vi "4p1_HW_Task2_gamagetd.vi"() -> ()   [LabVIEW 2016]
panel:
  out "Temperature T in C":dbl
  in  "Rois the resistance associated with the reference temperature in Ohm":dbl
  in  "Resistance r in Ohm":dbl
  in  "T-0 a reference temperature (in C)":dbl
  in  "ßis a thermal property of the materials (in K)":dbl
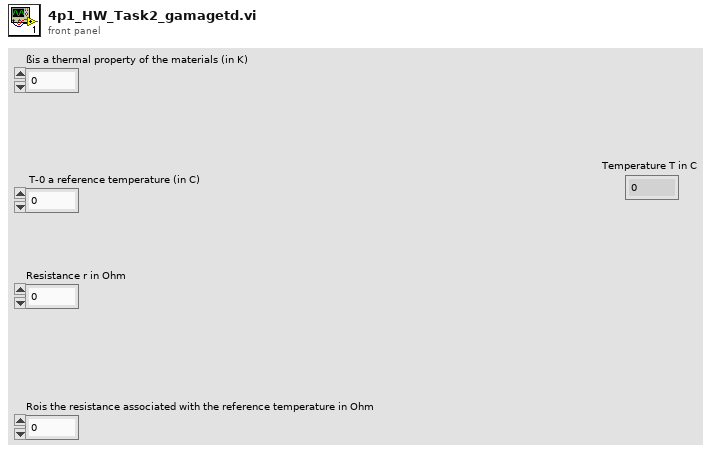
[diagram p1: front panel]
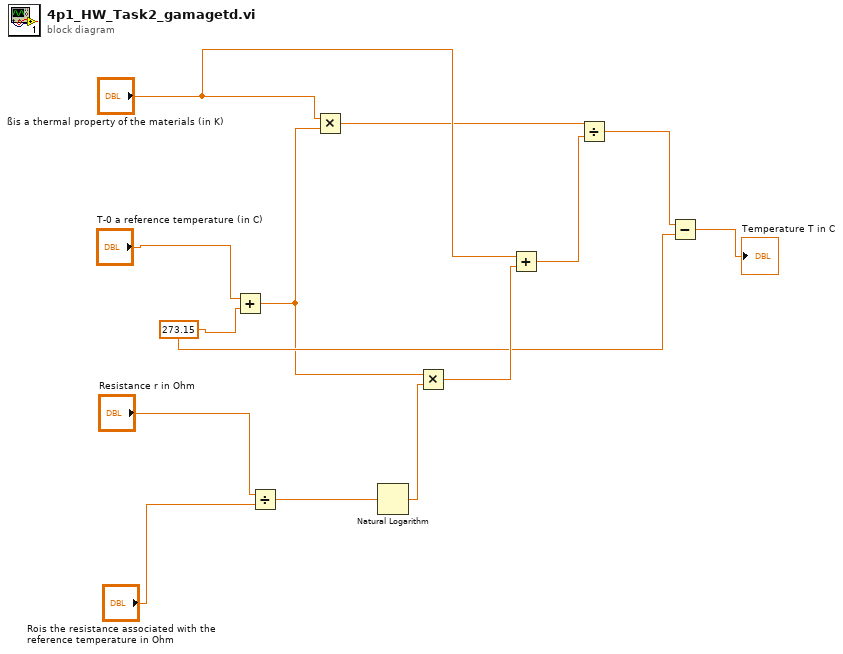
[diagram p0: block diagram]
diagram:
  w5 = 273.15
  n1 = Add(x="T-0 a reference temperature (in C)", y=w5) -> (x+y=w4:dbl)
  n2 = Divide(x="Resistance r in Ohm", y="Rois the resistance associated with the reference temperature in Ohm") -> (x/y=w12:dbl)
  n3 = Multiply(x="ßis a thermal property of the materials (in K)", y=w4) -> (x*y=w2:dbl)
  n4 = Natural Logarithm(1:w12) -> (0:w9:dbl)
  n5 = Multiply(x=w4, y=w9) -> (x*y=w8:dbl)
  n6 = Add(x="ßis a thermal property of the materials (in K)", y=w8) -> (x+y=w7:dbl)
  n7 = Divide(x=w2, y=w7) -> (x/y=w6:dbl)
  n8 = Subtract(x=w6, y=w5) -> (x-y=→"Temperature T in C":dbl)
